vi "set tracking state.vi"(6 "number of spots":u8, 7 "set state?":bool=TRUE, 8 "error in":errorcluster, 9 "tracking initializer":cluster{"x":i16, "y":i16, "z":i16}, 10 "spot number":u16, 11 "FPGA VI Reference In":T1) -> (0 "error out":errorcluster, 3 "FPGA VI Reference Out":T1)   [LabVIEW 2010]
uses:
  FPGA_ref.ctl
  <vilib>/rvi/interface/nirviReadWriteControl/nirviReadWriteControl.xnode
  <vilib>/rvi/interface/common/niFpgaNodeNameForErrorReporting.ctl
  <vilib>/rvi/errors/niLvFpgaWhatHappensToTopLevelVI.ctl
  <vilib>/Utility/error.llb/Error Cluster From Error Code.vi
  <vilib>/rvi/errors/niLvFpgaAdjustHostInterfaceError.vi
  NiFpgaLv.dll
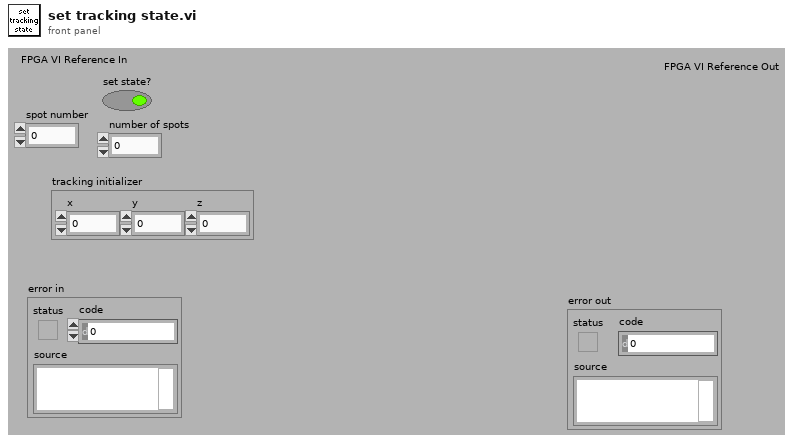
[diagram p1: front panel]
types:
  T1 = typedef "FPGA_ref.ctl" = refnum<k20>
  T2 = enum8{"no transition", "select state", "set state"}
  T3 = cluster{"x center":i16, "y center":i16, "z center":i16, "manual state selector":enum8{"no transition", "select state", "set state"}, "state number to set":u16}
  T4 = typedef "niFpgaNodeNameForErrorReporting.ctl" = enum16{"Open FPGA VI Reference", "Read/Write Control", "Invoke Method: Abort", "Invoke Method: Acknowledge IRQ", "Invoke Method: Download", "Invoke Method: FIFO.Configure", "Invoke Method: FIFO.Read", "Invoke Method: FIFO.Start", "Invoke Method: FIFO.Stop", "Invoke Method: FIFO.Write", "Invoke Method: Reset", "Invoke Method: Run", "Invoke Method: Wait on IRQ", "Close FPGA VI Reference"}
  T5 = typedef "niLvFpgaWhatHappensToTopLevelVI.ctl" = enum16{"top level VI scripted behind XNode", "top level VI inlined behind XNode"}
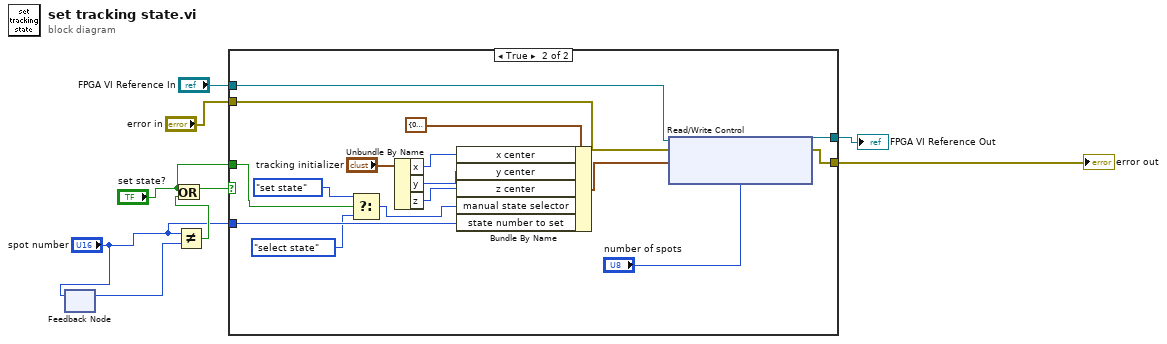
[diagram p0: block diagram]
diagram:
  n1 = feedback-in #1("spot number") -> ()
  n2 = feedback #1() -> (w5:u16)  [unwired: 1 in]
  n3 = Not Equal?(x="spot number", y=w5) -> (x != y?=w3:bool)
  n4 = Or(x="set state?", y=w3) -> (x .or. y?=w4:bool)
  n5 = case shown="True" w4 {
    tunnel: "FPGA VI Reference In" -> [w11 w23]
    tunnel: "error in" -> [w10 w22]
    tunnel: [w10 w21] -> w7
    tunnel: [w11 w20] -> w6
    tunnel: "spot number" -> [_ w16]
    tunnel: "set state?" -> [_ w14]
    frame False {
    }
    frame True {
      n6 = Select(t=T2."set state" ("manual state selector"), s=w14, f=T2."select state" ("manual state selector")) -> (s? t:f=w12:T2)
      n7 = Unbundle By Name("tracking initializer") -> ("x"=w26:i16, "y"=w25:i16, "z"=w24:i16)
      n8 = Bundle By Name(cluster=T3 {"x center"=0, "y center"=0, "z center"=0, "manual state selector"=enum."no transition", "state number to set"=0} ("Tracking State Initializer"), "x center"=w26, "y center"=w25, "z center"=w24, "manual state selector"=w12, "state number to set"=w16) -> (w18:T3)
      n9 = xnode "Read/Write Control"("FPGA VI Reference In"=w23, "error in"=w22, "Tracking State Initializer"=w18, "number of spots"="number of spots") -> ("FPGA VI Reference Out"=w20:T1, "error out"=w21:errorcluster)
    }
  }
  "FPGA VI Reference Out" <- w6
  "error out" <- w7
